vi "Calculate Zone.vi"(9 "Top Height":dbl, 10 "Bottom Height":dbl) -> (2 "Midpoint":dbl)   [LabVIEW 2018]
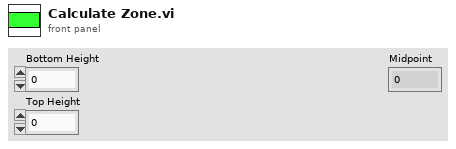
[diagram p1: front panel]
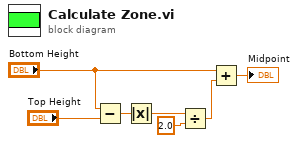
[diagram p0: block diagram]
diagram:
  n1 = Subtract(x="Bottom Height", y="Top Height") -> (x-y=w7:dbl)
  n2 = Absolute Value(x=w7) -> (abs(x)=w6:dbl)
  n3 = Divide(x=w6, y=2.0) -> (x/y=w5:dbl)
  n4 = Add(x="Bottom Height", y=w5) -> (x+y=→"Midpoint":dbl)
